vi "Create Antidoc HTML.vi"() -> ()   [LabVIEW 2021]
uses:
  <vilib>/Wovalab/AsciiDoc for LabVIEW/Output Format--enum.ctl
  <vilib>/Wovalab/AsciiDoc for LabVIEW/Wovalab_lib_AsciiDoctor.lvlib
  System.Windows.Forms
panel:
  in  "stop":bool
  in  "ADoc File":path=path "C:/Localdata/Projects/TriekselSoft/TriekselsoftApplicationFramework/Documentation/Project Documentation/Project.txt"
  in  "WebBrowser":refnum<k24>(container)
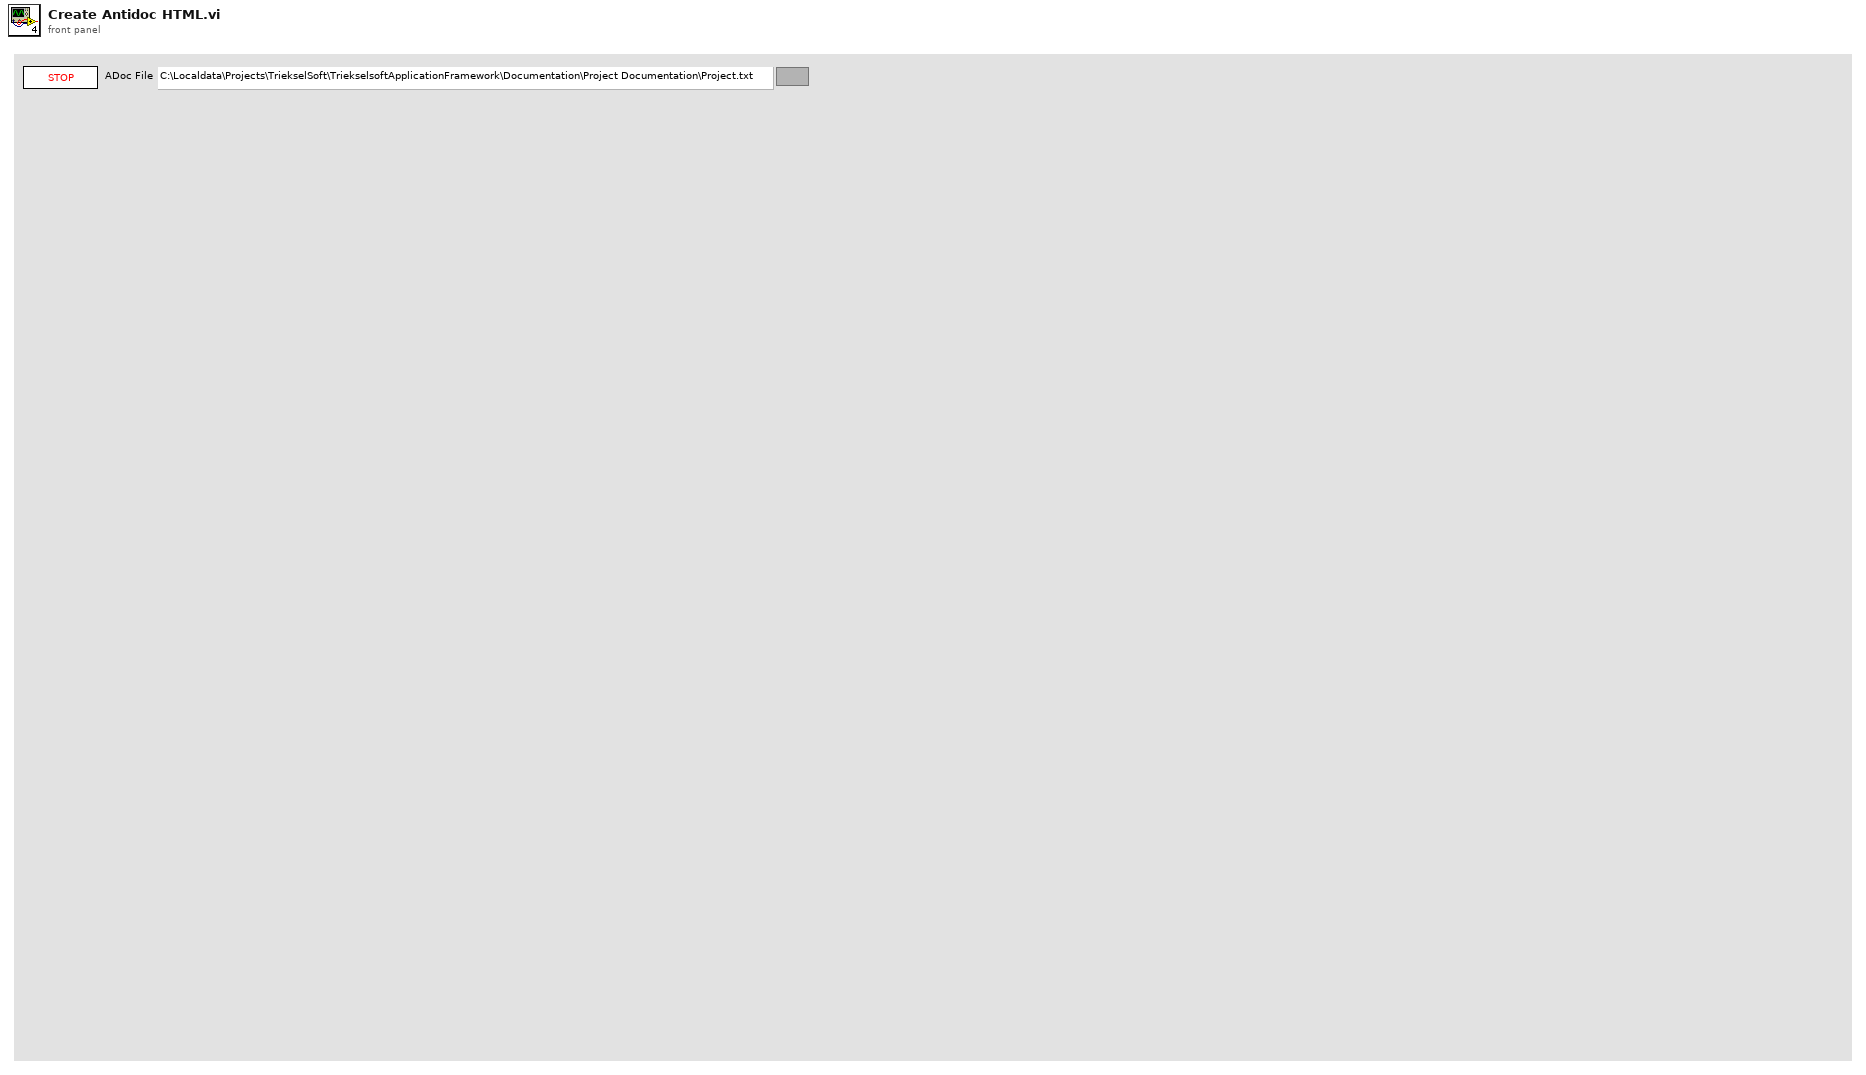
[diagram p1: front panel]
types:
  T1 = typedef "Wovalab_lib_AsciiDoctor.lvlib/Output Format--enum.ctl" = enum16{"HTML5", "PDF"}
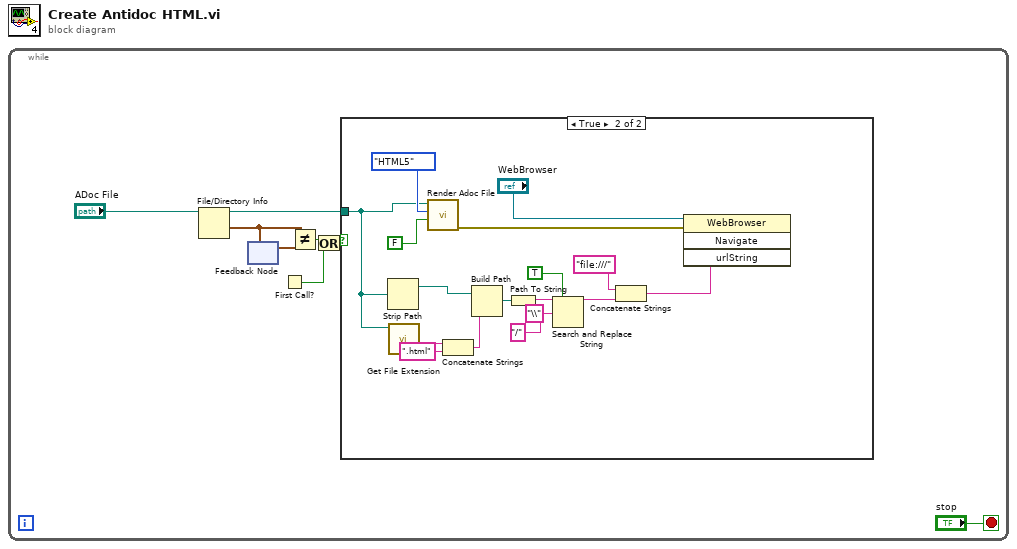
[diagram p0: block diagram]
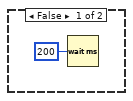
[diagram p2: hidden frame]
diagram:
  n1 = while {
    stop <- "stop" stop-if-true
    n2 = File/Directory Info(path="ADoc File") -> (path out=w7:path, last mod=w6:timestamp)  [unwired: 1 in, 5 out]
    n3 = feedback #1() -> (w5:timestamp)  [unwired: 1 in]
    n4 = feedback-in #1(w6) -> ()
    n5 = First Call?() -> (First Call?: T/F=w1:bool)
    n6 = Not Equal?(x=w6, y=w5) -> (x != y?=w4:bool)
    n7 = Or(x=w4, y=w1) -> (x .or. y?=w2:bool)
    n8 = case shown="True" w2 {
      tunnel: w7 -> [_ w22]
      frame False {
        n9 = Wait (ms)(milliseconds to wait=u32 200) -> ()  [unwired: 1 out]
      }
      frame True {
        n10 = Strip Path(path=w22) -> (stripped path=w21:path)  [unwired: 1 out]
        n11 = call <vilib>:"Get File Extension.vi"("file"=w22) -> ("filename without extension"=w20:string)  [unwired: 6 in, 4 out]
        n12 = call <vilib>:"Render Adoc File.vi"("Open Generated Document"=FALSE, "Output Format"=Output_Format--enum."HTML5", "Adoc File Path"=w22) -> ("error out"=w24:errorcluster)  [unwired: 6 in, 2 out]
        n13 = Concatenate Strings(w20, ".html" ("string")) -> (w18:string)
        n14 = Build Path(base path=w21, name or relative path=w18) -> (appended path=w17:path)
        n15 = Path To String(path=w17) -> (string=w16:string)
        n16 = Search and Replace String(replace all?=TRUE ("replace all? (F)"), input string=w16, search string="\\", replace string="/" ("search string")) -> (result string=w12:string)  [unwired: 4 in, 3 out]
        n17 = Concatenate Strings("file:///" ("string"), w12) -> (w10:string)
        n18 = invoke class="WebBrowser" method="Navigate"(reference="WebBrowser", error in=w24, "urlString"=w10) -> ()  [unwired: 1 in, 4 out]
      }
    }
  }
